vi "Convert Variant To Channel.vi"(8 "error in":errorcluster, 11 "Channel Variant":variant) -> (0 "error out":errorcluster, 3 "Channel Ref out":refnum<data-value>)   [LabVIEW 2024, in "Config File Parser.lvlib" / "Channel.lvclass"]
uses:
  Channel.lvclass
  Channel.lvclass/Channel.ctl
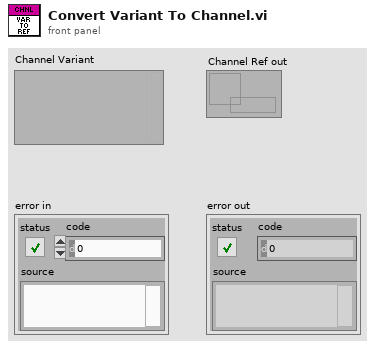
[diagram p1: front panel]
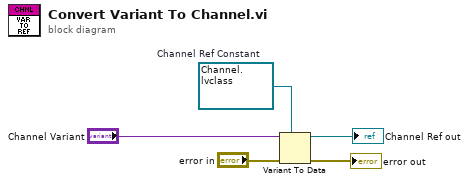
[diagram p0: block diagram]
diagram:
  w2 = refnum<data-value> refnum  # Channel Ref Constant
  n1 = Variant To Data(error in="error in", type=w2, Variant="Channel Variant") -> (data=→"Channel Ref out":refnum<data-value>, error out=→"error out":errorcluster)
